vi "hasPacketIdentifier.vi"(11 "UNSUBACK in":refnum<class "UNSUBACK.lvclass">) -> (2 "Has Packet Identifier":bool, 3 "UNSUBACK out":refnum<class "UNSUBACK.lvclass">)   [LabVIEW 2013, in "MQTT_Control_Packets.lvlib" / "UNSUBACK.lvclass"]
uses:
  UNSUBACK.lvclass
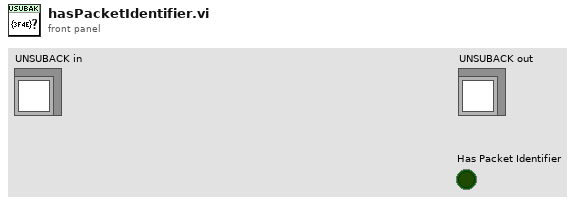
[diagram p1: front panel]
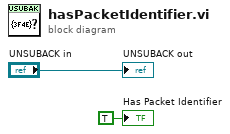
[diagram p0: block diagram]
diagram:
  "UNSUBACK out" <- "UNSUBACK in"
  "Has Packet Identifier" <- TRUE ("As Packet Identifier")
